vi "ReadData.vi"(8 "Error In":errorcluster, 11 "reference in":refnum<class "EncryptionDecorator.lvclass">) -> (0 "Error Out":errorcluster, 2 "Return(STRING)":string, 3 "reference in":refnum<class "EncryptionDecorator.lvclass">)   [LabVIEW 2020, in "EncryptionDecorator.lvclass"]
uses:
  EncryptionDecorator.lvclass
  DataSourceDecorator_class/DataSourceDecorator.lvclass
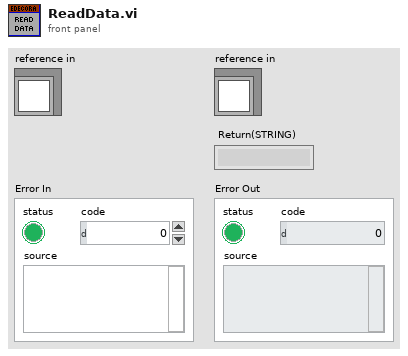
[diagram p1: front panel]
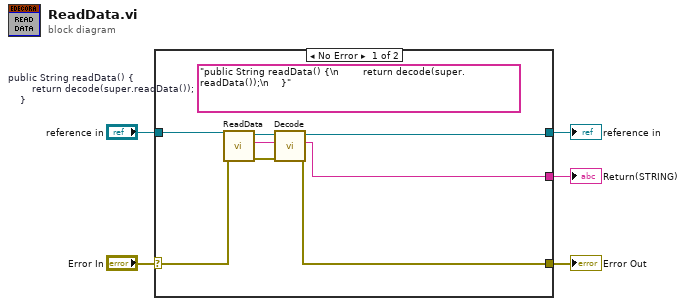
[diagram p0: block diagram]
diagram:
  n1 = case shown="No Error" "Error In" {
    selector: "Error In" -> [w12 w15]
    tunnel: [w8 w15] -> w4
    tunnel: [w7 w14] -> w2
    tunnel: "reference in" -> [w13 w14]
    tunnel: [w6 _] -> w1
    frame No Error {
      (unwired) "public String readData() {\n        return decode(super.readData());\n    }"  # public String readData() {         return decode(super.readData());     }
      n2 = call-parent "ReadData.vi"("Error In"=w12, "reference in"=w13) -> ("Error Out"=w11:errorcluster, "Return(STRING)"=w10:string, "reference out"=w9:refnum<class "EncryptionDecorator.lvclass">)  [unwired: 7 in]
      n3 = call "Decode.vi"("Error In"=w11, "Data"=w10, "reference in"=w9) -> ("Error Out"=w8:errorcluster, "Return(STRING)"=w6:string, "reference in"=w7:refnum<class "EncryptionDecorator.lvclass">)  [unwired: 6 in]
    }
    frame Error {
    }
  }
  "Error Out" <- w4
  "reference in" <- w2
  "Return(STRING)" <- w1
